vi "3D Parametric graph.vi"() -> (0 "Longitude out":dbl format="%.2f", 1 "Latitude out":dbl format="%.2f", 2 "3D graph out":refnum<k7>)   [LabVIEW 2013]
uses:
  <vilib>/Platform/NI_3dgraph.lvlib
panel:
  out "error out":errorcluster
  in  "3D Surface":refnum<k7>(container)
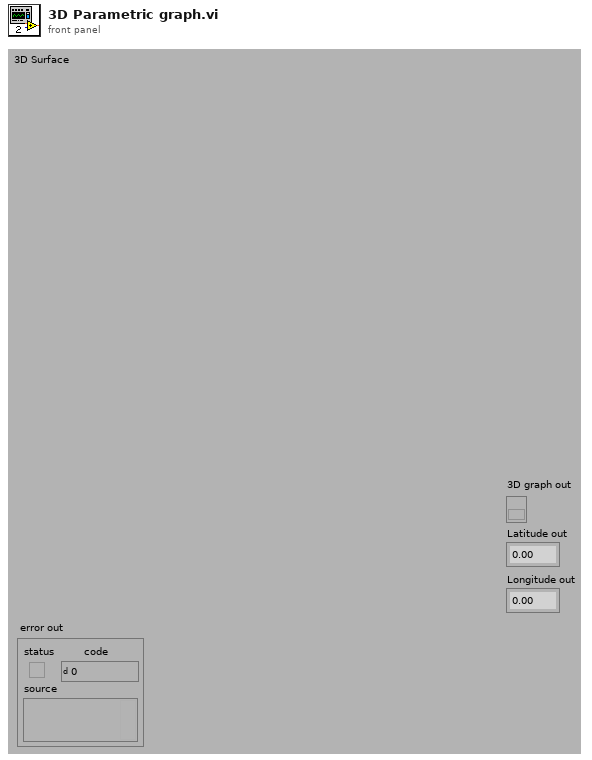
[diagram p1: front panel]
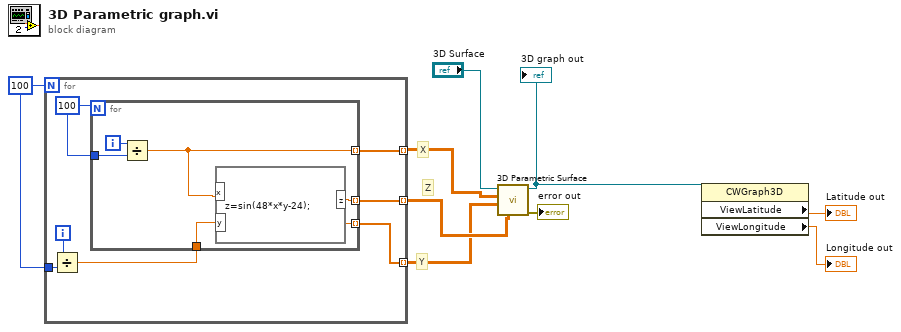
[diagram p0: block diagram]
diagram:
  w9 = 100
  # "Z"
  # "X"
  # "Y"
  n1 = for {
    N: w9 -> [_]
    tunnel: w9 -> [w14]
    tunnel: [w10] -> w2 mode=indexing
    tunnel: [w13] -> w4 mode=indexing
    tunnel: [w12] -> w3 mode=indexing
    i -> [w15]
    w16 = 100
    n2 = Divide(x=w15, y=w14) -> (x/y=w11:dbl)
    n3 = for {
      N: w16 -> [_]
      tunnel: w16 -> [w20]
      tunnel: [w19] -> w13 mode=indexing
      tunnel: w11 -> [w17]
      tunnel: [w18] -> w12 mode=indexing
      tunnel: [w17] -> w10 mode=indexing
      i -> [w21]
      n4 = Divide(x=w21, y=w20) -> (x/y=w19:dbl)
      n5 = formula code="z=sin(48*x*y-24);"("y"=w17, "x"=w19) -> ("z"=w18:dbl)
    }
  }
  n6 = call <vilib>:"3D Parametric Surface.vi"("z matrix"=w3, "y matrix"=w2, "x matrix"=w4, "3D graph"="3D Surface") -> ("error out"=→"error out":errorcluster, "3D graph out"=w5:refnum<k7>)  [unwired: 1 in, 5 out]
  "3D graph out" <- w5
  n7 = property class="CWGraph3D"(reference=w5) -> ("ViewLatitude"=→"Latitude out":dbl, "ViewLongitude"=→"Longitude out":dbl)  [unwired: 1 in, 2 out]
